vi "Byte Buffer.Mapping.Write Typed Array.vi"(0 "Byte Buffer in":refnum<class "Byte Buffer.lvclass">, 1 "data type":T1, 5 "buffer in":dbl[](array[numeric]), 7 "count":i32, 9 "buffer offset":i32, 11 "error in (no error)":errorcluster) -> (4 "Byte Buffer out":refnum<class "Byte Buffer.lvclass">, 6 "buffer out":dbl[](array[numeric]), 10 "new buffer offset":i32, 15 "error out":errorcluster)   [LabVIEW 2016, in "VeriStand Data.lvlib" / "Byte Buffer.lvclass"]
uses:
  Byte Buffer.lvclass
  Typedefs/Typedefs.Data Types.ctl
  Byte Buffer.lvclass/Byte Buffer.ctl
  Byte Buffer.Write (1D Boolean).vi
  Type Conversion/Type Conversion.From Double.Subset (1D Boolean).vi
  Byte Buffer.Write (1D SGL).vi
  Type Conversion/Type Conversion.From Double.Subset (1D SGL).vi
  Byte Buffer.Write (1D DBL).vi
  Byte Buffer.Write (1D I8).vi
  Type Conversion/Type Conversion.From Double.Subset (1D I8).vi
  Byte Buffer.Write (1D I16).vi
  Type Conversion/Type Conversion.From Double.Subset (1D I16).vi
  Byte Buffer.Write (1D I32).vi
  Type Conversion/Type Conversion.From Double.Subset (1D I32).vi
  Byte Buffer.Write (1D I64).vi
  Type Conversion/Type Conversion.From Double.Subset (1D I64).vi
  Byte Buffer.Write (1D U8).vi
  Type Conversion/Type Conversion.From Double.Subset (1D U8).vi
  Byte Buffer.Write (1D U16).vi
  Type Conversion/Type Conversion.From Double.Subset (1D U16).vi
  Byte Buffer.Write (1D U32).vi
  Type Conversion/Type Conversion.From Double.Subset (1D U32).vi
  Byte Buffer.Write (1D U64).vi
  Type Conversion/Type Conversion.From Double.Subset (1D U64).vi
  Type Conversion/Type Conversion.From Double.vi
  Type Conversion/Type Conversion.From Double (1D Boolean).vi
  Type Conversion/Type Conversion.From Double (1D SGL).vi
  Type Conversion/Type Conversion.From Double (1D I8).vi
  Type Conversion/Type Conversion.From Double (1D I16).vi
  Type Conversion/Type Conversion.From Double (1D I32).vi
  Type Conversion/Type Conversion.From Double (1D I64).vi
  Type Conversion/Type Conversion.From Double (1D U8).vi
  Type Conversion/Type Conversion.From Double (1D U16).vi
  Type Conversion/Type Conversion.From Double (1D U32).vi
  Type Conversion/Type Conversion.From Double (1D U64).vi
  SubVIs/Sizeof.Scalar.vi
  VeriStand Data.lvlib
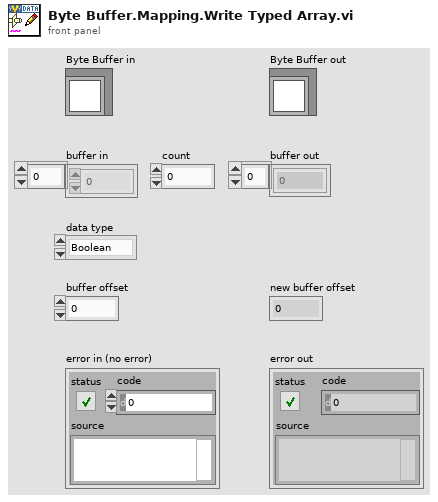
[diagram p1: front panel]
types:
  T1 = typedef "VeriStand Data.lvlib/Typedefs.Data Types.ctl" = enum16{"Boolean", "Single", "Double", "I8", "I16", "I32", "I64", "U8", "U16", "U32", "U64"}
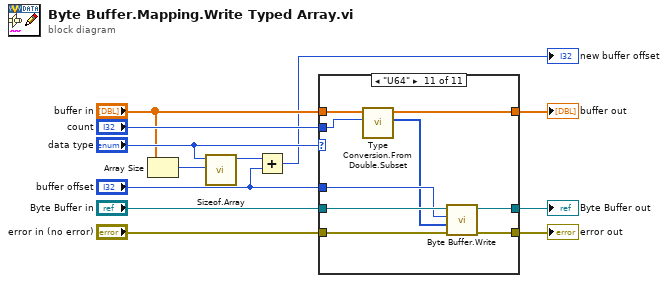
[diagram p0: block diagram]
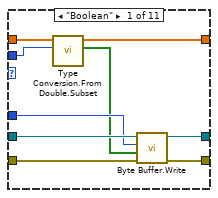
[diagram p2: hidden frame]
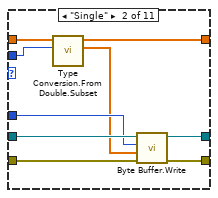
[diagram p3: hidden frame]
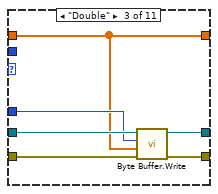
[diagram p4: hidden frame]
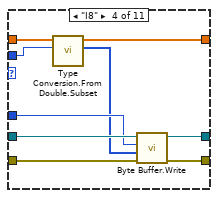
[diagram p5: hidden frame]
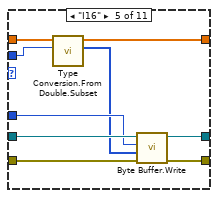
[diagram p6: hidden frame]
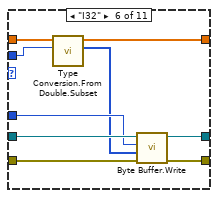
[diagram p7: hidden frame]
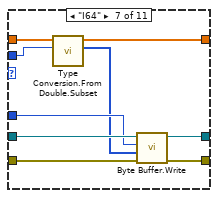
[diagram p8: hidden frame]
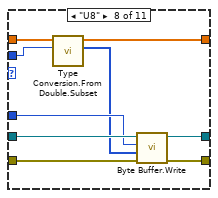
[diagram p9: hidden frame]
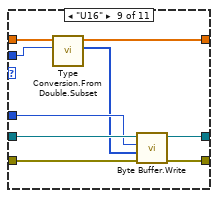
[diagram p10: hidden frame]
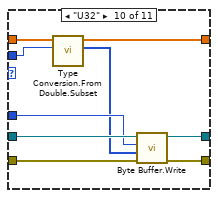
[diagram p11: hidden frame]
diagram:
  n1 = Array Size(array="buffer in") -> (size(s)=w9:i32)
  n2 = call "Sizeof.Array.vi"("count"=w9, "data type"="data type") -> ("size"=w4:i32)  [unwired: 9 in]
  n3 = Add(x=w4, y="buffer offset") -> (x+y=→"new buffer offset":i32)
  n4 = case shown="\"U64\"" "data type" {
    tunnel: "buffer in" -> [w21 w30 w31 w45 w54 w63 w72 w81 w90 w99 w108]
    tunnel: "buffer offset" -> [w18 w27 w34 w42 w51 w60 w69 w78 w87 w96 w105]
    tunnel: "Byte Buffer in" -> [w20 w29 w36 w44 w53 w62 w71 w80 w89 w98 w107]
    tunnel: [w19 w28 w35 w43 w52 w61 w70 w79 w88 w97 w106] -> w12
    tunnel: "error in (no error)" -> [w17 w26 w33 w41 w50 w59 w68 w77 w86 w95 w104]
    tunnel: [w16 w25 w32 w40 w49 w58 w67 w76 w85 w94 w103] -> w10
    tunnel: [w15 w24 w31 w39 w48 w57 w66 w75 w84 w93 w102] -> w7
    tunnel: "count" -> [w14 w23 _ w38 w47 w56 w65 w74 w83 w92 w101]
    frame "Boolean" {
      n5 = call-poly "Type Conversion.From Double.Subset.vi"("count"=w14, "values in"=w21) -> ("converted values out"=w13:bool[], "values out"=w15:dbl[])  [unwired: 8 in]
      n6 = call-poly "Byte Buffer.Write.vi"("error in (no error)"=w17, "values"=w13, "buffer offset"=w18, "Byte Buffer in"=w20) -> ("error out"=w16:errorcluster, "Byte Buffer out"=w19:refnum<class "Byte Buffer.lvclass">)  [unwired: 6 in]
    }
    frame "Single" {
      n7 = call-poly "Type Conversion.From Double.Subset.vi"("count"=w23, "values in"=w30) -> ("converted values out"=w22:sgl[], "values out"=w24:dbl[])  [unwired: 8 in]
      n8 = call-poly "Byte Buffer.Write.vi"("error in (no error)"=w26, "values"=w22, "buffer offset"=w27, "Byte Buffer in"=w29) -> ("error out"=w25:errorcluster, "Byte Buffer out"=w28:refnum<class "Byte Buffer.lvclass">)  [unwired: 6 in]
    }
    frame "Double" {
      n9 = call-poly "Byte Buffer.Write.vi"("error in (no error)"=w33, "values"=w31, "buffer offset"=w34, "Byte Buffer in"=w36) -> ("error out"=w32:errorcluster, "Byte Buffer out"=w35:refnum<class "Byte Buffer.lvclass">)  [unwired: 6 in]
    }
    frame "I8" {
      n10 = call-poly "Type Conversion.From Double.Subset.vi"("count"=w38, "values in"=w45) -> ("converted values out"=w37:i8[], "values out"=w39:dbl[])  [unwired: 8 in]
      n11 = call-poly "Byte Buffer.Write.vi"("error in (no error)"=w41, "values"=w37, "buffer offset"=w42, "Byte Buffer in"=w44) -> ("error out"=w40:errorcluster, "Byte Buffer out"=w43:refnum<class "Byte Buffer.lvclass">)  [unwired: 6 in]
    }
    frame "I16" {
      n12 = call-poly "Type Conversion.From Double.Subset.vi"("count"=w47, "values in"=w54) -> ("converted values out"=w46:i16[], "values out"=w48:dbl[])  [unwired: 8 in]
      n13 = call-poly "Byte Buffer.Write.vi"("error in (no error)"=w50, "values"=w46, "buffer offset"=w51, "Byte Buffer in"=w53) -> ("error out"=w49:errorcluster, "Byte Buffer out"=w52:refnum<class "Byte Buffer.lvclass">)  [unwired: 6 in]
    }
    frame "I32" {
      n14 = call-poly "Type Conversion.From Double.Subset.vi"("count"=w56, "values in"=w63) -> ("converted values out"=w55:i32[], "values out"=w57:dbl[])  [unwired: 8 in]
      n15 = call-poly "Byte Buffer.Write.vi"("error in (no error)"=w59, "values"=w55, "buffer offset"=w60, "Byte Buffer in"=w62) -> ("error out"=w58:errorcluster, "Byte Buffer out"=w61:refnum<class "Byte Buffer.lvclass">)  [unwired: 6 in]
    }
    frame "I64" {
      n16 = call-poly "Type Conversion.From Double.Subset.vi"("count"=w65, "values in"=w72) -> ("converted values out"=w64:i64[], "values out"=w66:dbl[])  [unwired: 8 in]
      n17 = call-poly "Byte Buffer.Write.vi"("error in (no error)"=w68, "values"=w64, "buffer offset"=w69, "Byte Buffer in"=w71) -> ("error out"=w67:errorcluster, "Byte Buffer out"=w70:refnum<class "Byte Buffer.lvclass">)  [unwired: 6 in]
    }
    frame "U8" {
      n18 = call-poly "Type Conversion.From Double.Subset.vi"("count"=w74, "values in"=w81) -> ("converted values out"=w73:u8[], "values out"=w75:dbl[])  [unwired: 8 in]
      n19 = call-poly "Byte Buffer.Write.vi"("error in (no error)"=w77, "values"=w73, "buffer offset"=w78, "Byte Buffer in"=w80) -> ("error out"=w76:errorcluster, "Byte Buffer out"=w79:refnum<class "Byte Buffer.lvclass">)  [unwired: 6 in]
    }
    frame "U16" {
      n20 = call-poly "Type Conversion.From Double.Subset.vi"("count"=w83, "values in"=w90) -> ("converted values out"=w82:u16[], "values out"=w84:dbl[])  [unwired: 8 in]
      n21 = call-poly "Byte Buffer.Write.vi"("error in (no error)"=w86, "values"=w82, "buffer offset"=w87, "Byte Buffer in"=w89) -> ("error out"=w85:errorcluster, "Byte Buffer out"=w88:refnum<class "Byte Buffer.lvclass">)  [unwired: 6 in]
    }
    frame "U32" {
      n22 = call-poly "Type Conversion.From Double.Subset.vi"("count"=w92, "values in"=w99) -> ("converted values out"=w91:u32[], "values out"=w93:dbl[])  [unwired: 8 in]
      n23 = call-poly "Byte Buffer.Write.vi"("error in (no error)"=w95, "values"=w91, "buffer offset"=w96, "Byte Buffer in"=w98) -> ("error out"=w94:errorcluster, "Byte Buffer out"=w97:refnum<class "Byte Buffer.lvclass">)  [unwired: 6 in]
    }
    frame "U64" {
      n24 = call-poly "Type Conversion.From Double.Subset.vi"("count"=w101, "values in"=w108) -> ("converted values out"=w100:u64[], "values out"=w102:dbl[])  [unwired: 8 in]
      n25 = call-poly "Byte Buffer.Write.vi"("error in (no error)"=w104, "values"=w100, "buffer offset"=w105, "Byte Buffer in"=w107) -> ("error out"=w103:errorcluster, "Byte Buffer out"=w106:refnum<class "Byte Buffer.lvclass">)  [unwired: 6 in]
    }
  }
  "error out" <- w10
  "Byte Buffer out" <- w12
  "buffer out" <- w7
